vi "analog_ramp_block.vi"() -> ()   [LabVIEW 2017]
uses:
  <vilib>/eio/EIONode/EIONode.xnode
  <vilib>/rvi/eio/common/nirviEmuTemplateMethod_errors.vi
panel:
  out "Tick Count(Ticks)":u32
  out "x/y":fxp<+/-,32,9>
  out "elapsed time":i16(graph)
  out "AO":i16(graph)
  out "ctr1":i32
  out "x-y":i32
  out "error [A]":fxp<+/-,64,33>
  in  "init I":fxp<+,32,8>
  out "AO":fxp<+,47,23>
  out "error":fxp<+/-,33,9>
  in  "ramp time [10*us] 2":fxp<+,16,16>
  in  "finalI":fxp<+,32,8>
  out "It":fxp<+,32,8>
  out "elapsed time 2":fxp<+,32,18>
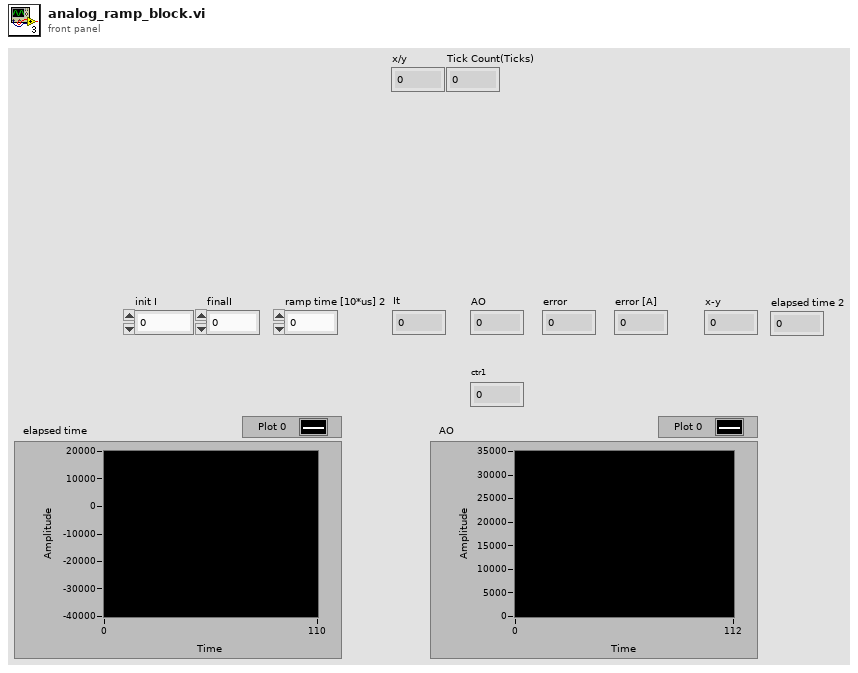
[diagram p1: front panel]
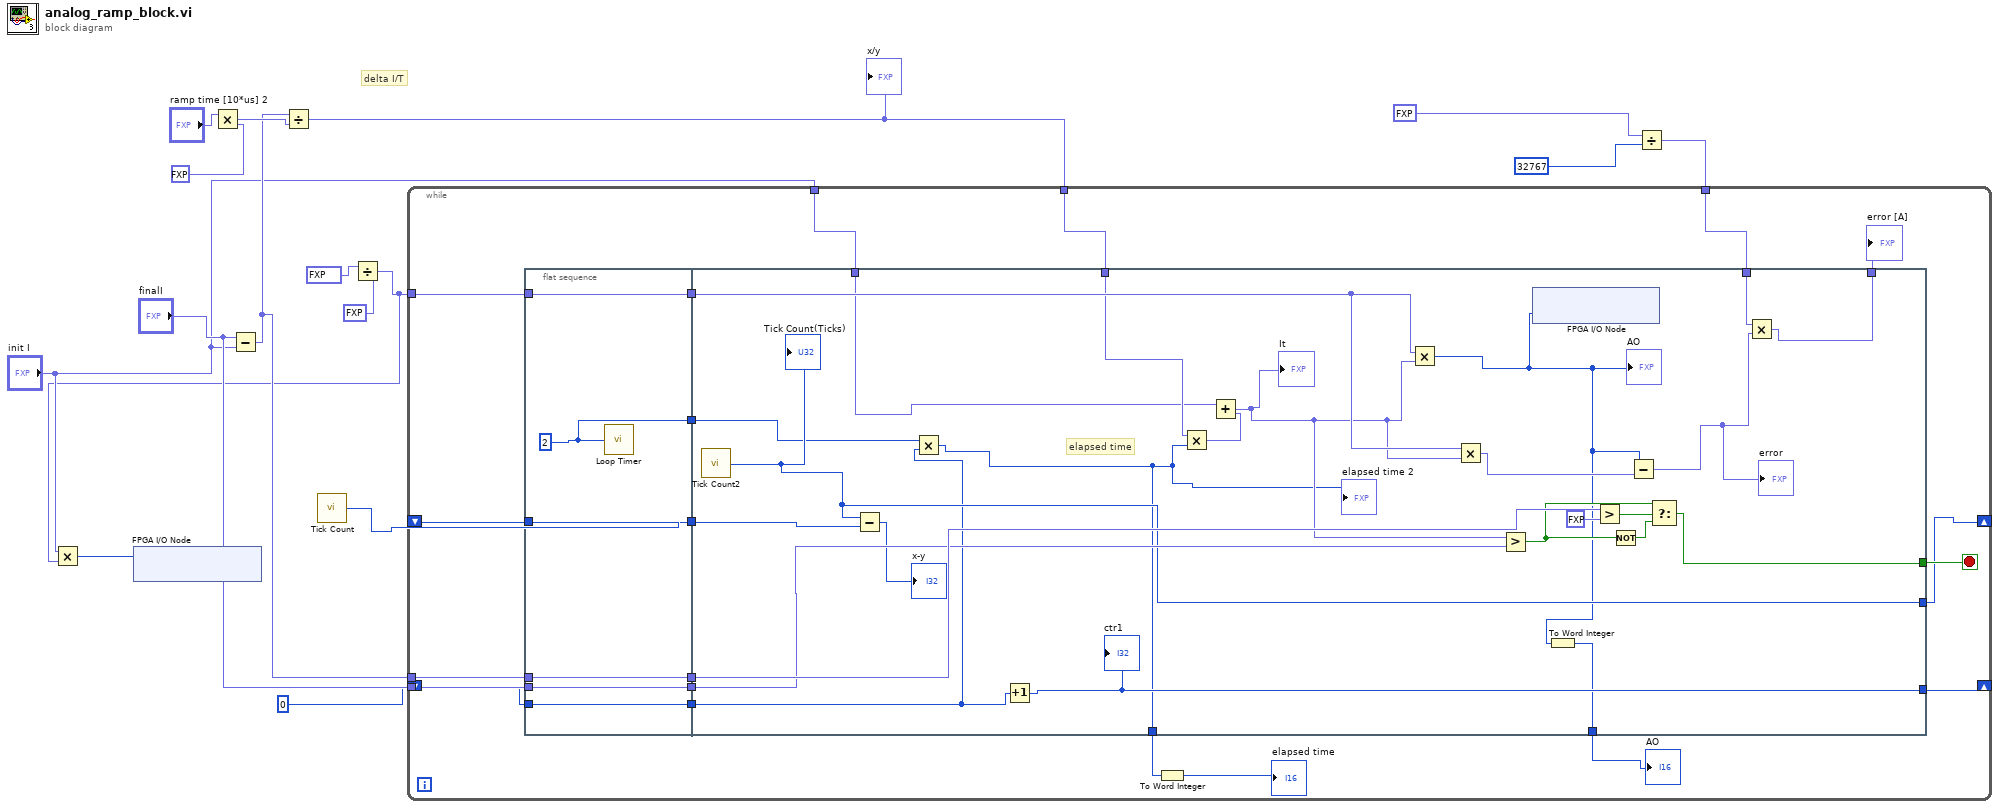
[diagram p0: block diagram]
diagram:
  # "delta I/T"
  n1 = Multiply(x="ramp time [10*us] 2", y=fxp<+,16,16> 10.0) -> (x*y=w11:fxp<+,32,32>)
  n2 = Subtract(x="finalI", y="init I") -> (x-y=w9:fxp<+/-,32,9>)
  n3 = Divide(x=w9, y=w11) -> (x/y=w10:fxp<+/-,32,9>)
  "x/y" <- w10
  n4 = call "Tick Count"() -> ("Tick Count(Ticks)"=w14:u32)
  n5 = Divide(x=fxp<+,15,15> 32767.0, y=fxp<+,6,8> 220.0) -> (x/y=w1:fxp<+,15,15>)
  n6 = Multiply(x="init I", y=w1) -> (x*y=w3:i16)
  n7 = xnode "FPGA I/O Node"("Connector0/AO7"=w3) -> ()  [unwired: 1 in, 1 out]
  n8 = Divide(x=fxp<+,15,15> 220.0, y=i16 32767) -> (x/y=w5:fxp<+,32,16>)
  n9 = while {
    shift-right: [w28] -> _
    shift-left: w14 -> [w36]
    tunnel: w1 -> [w37]
    tunnel: w10 -> [w34]
    tunnel: "init I" -> [w33]
    tunnel: w9 -> [w32]
    tunnel: "finalI" -> [w31]
    tunnel: w5 -> [w30]
    shift-right: [w21] -> _
    shift-left: i16 0 -> [w22]
    stop <- w35 stop-if-true
    n10 = flat-sequence {
      tunnel: w31 -> [w40]
      tunnel: w32 -> [w41]
      tunnel: w36 -> [w42]
      tunnel: w37 -> [w43]
      tunnel: [w43] -> w27
      tunnel: [w42] -> w26
      tunnel: [w41] -> w25
      tunnel: [w40] -> w24
      tunnel: [w39] -> w23
      tunnel: w22 -> [w39]
      tunnel: [w38] -> w17
      tunnel: [w66] -> w35
      tunnel: w34 -> [w65]
      tunnel: w33 -> [w64]
      tunnel: w30 -> [w53]
      tunnel: [w52] -> w29
      tunnel: [w50] -> w28
      tunnel: w27 -> [w68]
      tunnel: w26 -> [w67]
      tunnel: w25 -> [w63]
      tunnel: w24 -> [w62]
      tunnel: w23 -> [w46]
      tunnel: [w49] -> w21
      tunnel: [w47] -> w20
      tunnel: [w44] -> w18
      tunnel: w17 -> [w45]
      frame #0 {
        w38 = u32 2 ("Count(uSec)")
        n11 = call "Loop Timer"("Count(uSec)"=w38) -> ()  [unwired: 1 out]
      }
      frame #1 {
        # "elapsed time"
        n12 = call "Tick Count2"() -> ("Tick Count(Ticks)"=w50:u32)
        "Tick Count(Ticks)" <- w50
        n13 = Subtract(x=w50, y=w67) -> (x-y=→"x-y":i32)
        n14 = Multiply(x=w45, y=w46) -> (x*y=w44:u32)
        "elapsed time 2" <- w44
        n15 = Increment(x=w46) -> (x+1=w49:i32)
        "ctr1" <- w49
        n16 = Multiply(x=w65, y=w44) -> (x*y=w60:fxp<+/-,32,9>)
        n17 = Add(x=w64, y=w60) -> (x+y=w56:fxp<+,32,8>)
        "It" <- w56
        n18 = Multiply(x=w68, y=w56) -> (x*y=w48:i16)
        "AO" <- w48
        n19 = Multiply(x=w68, y=w56) -> (x*y=w61:fxp<+,32,15>)
        n20 = Greater?(x=w56, y=w62) -> (0:w55:bool)
        n21 = xnode "FPGA I/O Node"("Connector0/AO7"=w48) -> ()  [unwired: 1 in, 1 out]
        n22 = To Word Integer(number=w48) -> (16bit integer=w47:i16)
        n23 = Greater?(x=w63, y=fxp<+/-,31,9> 0.0) -> (0:w57:bool)
        n24 = Not(x=w55) -> (.not. x?=w54:bool)
        n25 = Subtract(x=w48, y=w61) -> (x-y=w59:fxp<+/-,32,16>)
        "error" <- w59
        n26 = Select(t=w55, s=w57, f=w54) -> (s? t:f=w66:bool)
        n27 = Multiply(x=w53, y=w59) -> (x*y=w52:fxp<+,32,16>)
      }
    }
    n28 = To Word Integer(number=w18) -> (16bit integer=→"elapsed time":i16)
    "error [A]" <- w29
    "AO" <- w20
  }
